vi "MotorFwd_1.vi"   [LabVIEW 2012]
uses:
  <vilib>/NXT/Subs/MotorOutput.ctl
types:
  T1 = typedef "MotorOutput.ctl" = u8
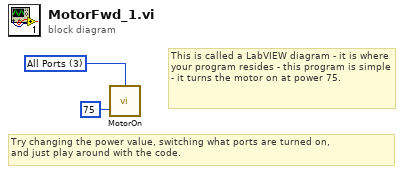
[diagram p0: block diagram]
diagram:
  w2 = T1 3 items=["Port A"=0, "Port B"=1, "Port C"=2, "Ports A & B"=4, "Ports A & C"=5, "Ports B & C"=6, "All Ports"=3] ("Output Port (All Ports)")
  # "Try changing the power value, switching what ports are turned on,\nand just play around with the code."
  # "This is called a LabVIEW diagram - it is where your program resides - this program is simple - it turns the motor on at power 75."
  n1 = call <vilib>:"MotorOn.vi"("Power (75)"=75, "Output Port (All Ports)"=w2) -> ()  [unwired: 2 in, 1 out]
